vi "Write Sweep Rate.vi"(8 "error in (no error)":errorcluster, 10 "rate":dbl[unit] caption="Rate", 11 "Power Supply in":refnum<class "Power Supply.lvclass">) -> (0 "error out":errorcluster, 3 "Power Supply out":refnum<class "Power Supply.lvclass">)   [LabVIEW 2009, in "Power Supply.lvclass"]
uses:
  Power Supply.lvclass
  Power Supply.lvclass/Power Supply.ctl
panel:
  out "rateok":bool
  out "maxrate":dbl[unit]
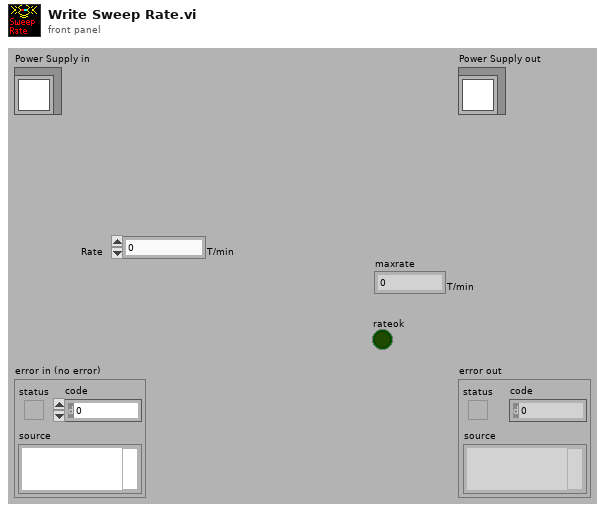
[diagram p1: front panel]
types:
  T1 = typedef "PSIO.ctl" = cluster{"Address":T2, "Version":enum16{"PS", "IPS"}}
  T2 = typedef "OxfordAddress.ctl" = cluster{"Com Port":i32, "ISOBUS Address":i32, "GPIB Address":i16, "Communication":enum16{"RS232", "ISOBUS", "GPIB", "Gateway"}}
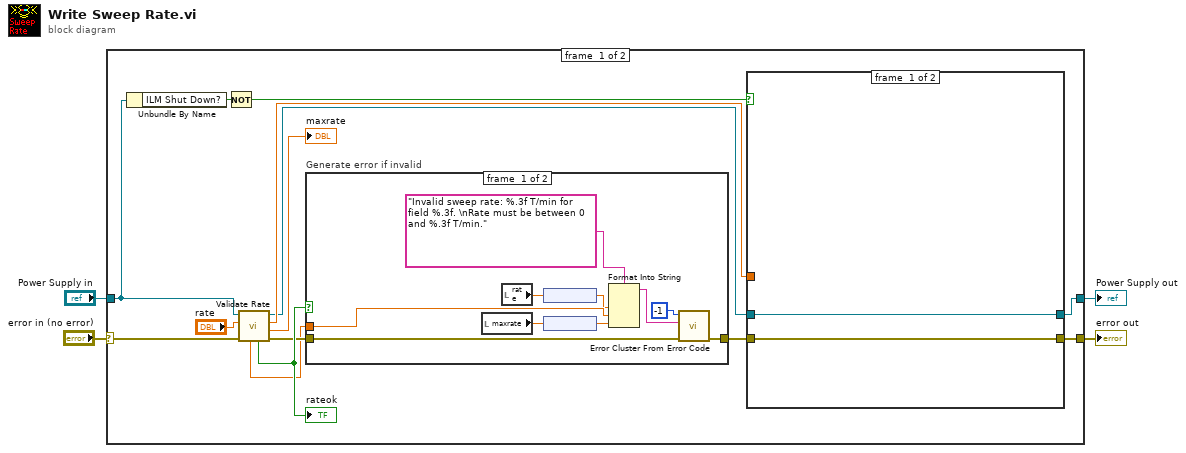
[diagram p0: block diagram]
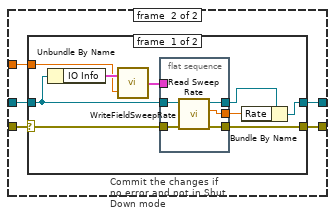
[diagram p2: hidden frame]
diagram:
  n1 = case shown="No Error" "error in (no error)" {
    selector: "error in (no error)" -> [w14 w53]
    tunnel: [w18 w54] -> w1
    tunnel: [w15 w53] -> w2
    tunnel: "Power Supply in" -> [w7 w54]
    frame #0 {
      n2 = Unbundle By Name(w7) -> ("ILM Shut Down?"=w6:bool)
      n3 = Not(x=w6) -> (.not. x?=w5:bool)
      n4 = call "Validate Rate.vi"("error IO"=w14, "rate"="rate", "Power Supply in"=w7) -> ("error out"=w13:errorcluster, "Max rate"=→"maxrate":dbl[unit], "Coerced rate"=w9:dbl[unit], "Power Supply out"=w8:refnum<class "Power Supply.lvclass">, "Coerced?"=w16:bool, "Field"=w12:dbl[unit])  [unwired: 3 in]
      "rateok" <- w16
      n5 = case "Generate error if invalid" shown="False" w16 {
        tunnel: [w51 w52] -> w17
        tunnel: w13 -> [w47 w52]
        tunnel: w12 -> [w45 _]
        frame #0 {
          n6 = local read "maxrate"() -> (w46:dbl[unit])
          n7 = local read "rate"() -> (w44:dbl[unit])
          n8 = node(w44) -> (w43:dbl)
          n9 = node(w46) -> (w42:dbl)
          n10 = Format Into String(format string="Invalid sweep rate: %.3f T/min for field %.3f. \nRate must be between 0 and %.3f T/min.", w43, w45, w42) -> (resulting string=w49:string)  [unwired: 2 in, 1 out]
          n11 = call <vilib>:"Error Cluster From Error Code.vi"("error in (no error)"=w47, "error message (\"\")"=w49, "error code (0)"=-1) -> ("error out"=w51:errorcluster)  [unwired: 6 in]
        }
        frame #1 {
        }
      }
      n12 = case shown="True" w5 {
        tunnel: [w20 w25] -> w18
        tunnel: w17 -> [w19 w24]
        tunnel: [w19 w23] -> w15
        tunnel: w9 -> [_ w22]
        tunnel: w8 -> [w20 w21]
        frame #0 {
        }
        frame #1 {
          n13 = case "Commit the changes if no error and not in Shut Down mode" shown="No Error" w24 {
            selector: w24 -> [w27 w41]
            tunnel: w22 -> [w32 _]
            tunnel: [w26 w41] -> w23
            tunnel: w21 -> [w30 w40]
            tunnel: [w33 w40] -> w25
            frame #0 {
              n14 = Unbundle By Name(w30) -> ("IO Info"=w34:T1)
              n15 = call "WriteFieldSweepRate.vi"("Sweep rate"=w32, "IO Info"=w34) -> ("IO Info"=w28:T1)
              n16 = flat-sequence {
                tunnel: [w39] -> w31
                tunnel: w30 -> [w38]
                tunnel: [w37] -> w29
                tunnel: w28 -> [_]
                tunnel: w27 -> [w36]
                tunnel: [w35] -> w26
                frame #0 {
                  n17 = call-dynamic "Read Sweep Rate.vi"("error in (no error)"=w36, "Power Supply in"=w38) -> ("error out"=w35:errorcluster, "Field sweep rate"=w39:dbl[unit], "Power Supply out"=w37:refnum<class "Power Supply.lvclass">)  [unwired: 7 in]
                }
              }
              n18 = Bundle By Name(cluster=w29, "Rate"=w31) -> (w33:refnum<class "Power Supply.lvclass">)
            }
            frame #1 {
            }
          }
        }
      }
    }
    frame #1 {
    }
  }
  "Power Supply out" <- w1
  "error out" <- w2
